vi "read config.vi"(8 "error in (no error)":errorcluster, 10 "config file path":path, 11 "controller in":refnum<class "controller.lvclass">) -> (0 "error out":errorcluster, 3 "controller out":refnum<class "controller.lvclass">)   [LabVIEW 2025, in "controller.lvclass"]
uses:
  controller.lvclass
  controller.lvclass/controller.ctl
  36d25bd7-cc9f-45b5-8260-26248bae390a.vi
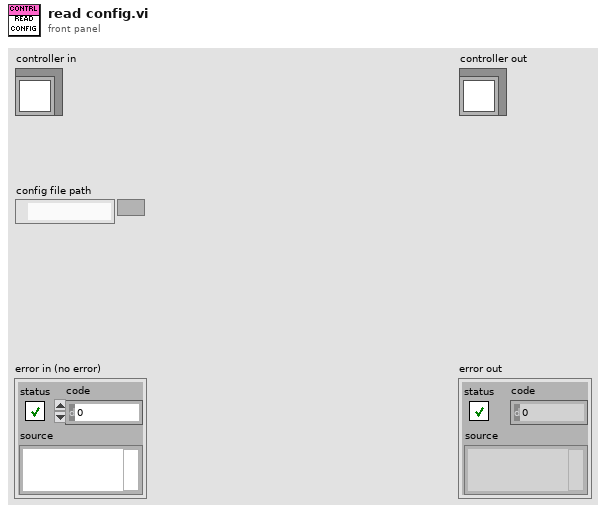
[diagram p1: front panel]
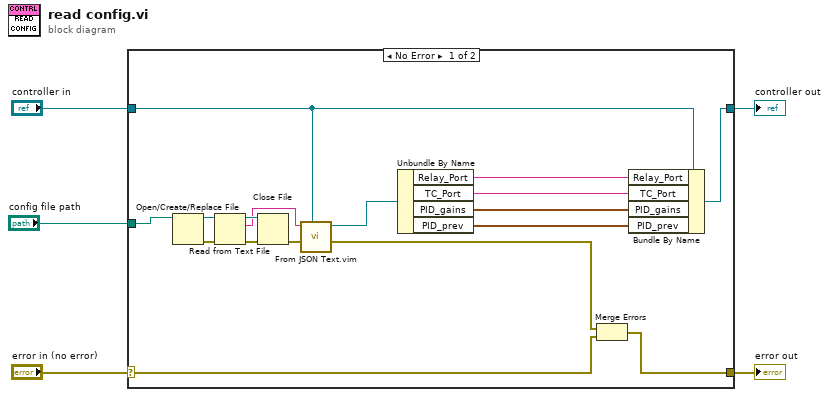
[diagram p0: block diagram]
diagram:
  n1 = case shown="No Error" "error in (no error)" {
    selector: "error in (no error)" -> [w12 w24]
    tunnel: [w11 w24] -> w4
    tunnel: [w6 w23] -> w2
    tunnel: "controller in" -> [w10 w23]
    tunnel: "config file path" -> [w13 _]
    frame No Error {
      n2 = Open/Create/Replace File(file path (use dialog)=w13) -> (refnum out=w19:refnum<file>, error out=w22:errorcluster)  [unwired: 5 in, 1 out]
      n3 = Read from Text File(file (use dialog)=w19, error in=w22) -> (refnum out=w20:refnum<file>, text=w18:string, error out=w21:errorcluster)  [unwired: 2 in, 1 out]
      n4 = Close File(refnum=w20, error in=w21) -> (error out=w17:errorcluster)  [unwired: 1 out]
      n5 = call "From JSON Text.vim"("Data Type and Default Value"=w10, "error in (no error)"=w17, "JSON"=w18) -> ("error out"=w16:errorcluster, "Data out"=w15:refnum<class "controller.lvclass">)  [unwired: 7 in]
      n6 = Unbundle By Name(w15) -> ("Relay_Port"=w9:string, "TC_Port"=w8:string, "PID_gains"=w7:cluster{"P":dbl, "I":dbl, "D":dbl}, "PID_prev"=w14:cluster{"e_prev":dbl, "e_int":dbl})
      n7 = Merge Errors(w16, w12) -> (w11:errorcluster)
      n8 = Bundle By Name(cluster=w10, "Relay_Port"=w9, "TC_Port"=w8, "PID_gains"=w7, "PID_prev"=w14) -> (w6:refnum<class "controller.lvclass">)
    }
    frame Error {
    }
  }
  "error out" <- w4
  "controller out" <- w2
